vi "Get SLSC Module By Slot.vi"(8 "error in (no error)":errorcluster, 10 "Slot":u32=1, 11 "SLSC Chassis":u64) -> (0 "error out":errorcluster, 2 "SLSC Module":u64, 3 "SLSC Chassis out":u64)   [LabVIEW 2020, in "VeriStand SLSC Scripting.lvlib"]
uses:
  VeriStand SLSC Scripting.lvlib
  NationalInstruments.VeriStand.SystemDefinitionAPI
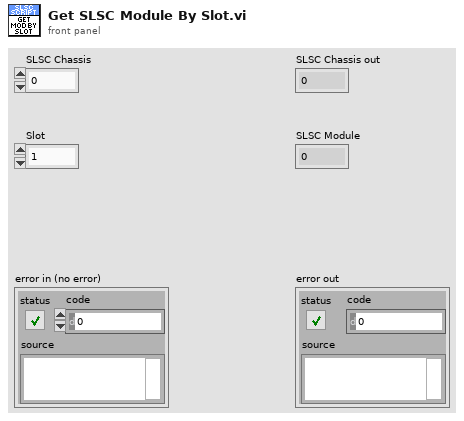
[diagram p1: front panel]
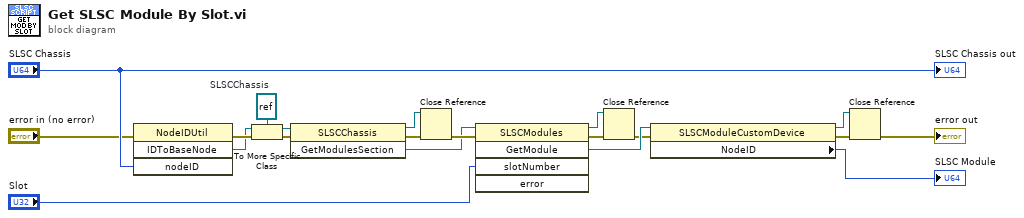
[diagram p0: block diagram]
diagram:
  w14 = refnum<k24> refnum  # SLSCChassis
  n1 = invoke class="NodeIDUtil" method="IDToBaseNode"(error in="error in (no error)", "nodeID"="SLSC Chassis") -> (error out=w11:errorcluster, "IDToBaseNode"=w10:refnum<k24>)  [unwired: 2 in, 2 out]
  n2 = To More Specific Class(target class=w14, reference=w10, error in=w11) -> (specific class reference=w12:refnum<k24>, error out=w13:errorcluster)
  n3 = invoke class="SLSCChassis" method="GetModulesSection"(reference=w12, error in=w13) -> (reference out=w7:refnum<k24>, error out=w9:errorcluster, "GetModulesSection"=w6:refnum<k24>)  [unwired: 1 in]
  n4 = Close Reference(reference=w7, error in (no error)=w9) -> (error out=w18:errorcluster)
  n5 = invoke class="SLSCModules" method="GetModule"(reference=w6, error in=w18, "slotNumber"="Slot") -> (reference out=w1:refnum<k24>, error out=w8:errorcluster, "GetModule"=w4:refnum<k24>)  [unwired: 2 in, 2 out]
  n6 = Close Reference(reference=w1, error in (no error)=w8) -> (error out=w2:errorcluster)
  n7 = property class="SLSCModuleCustomDevice"(reference=w4, error in=w2) -> (reference out=w3:refnum<k24>, error out=w17:errorcluster, "NodeID"=→"SLSC Module":u64)
  n8 = Close Reference(reference=w3, error in (no error)=w17) -> (error out=→"error out":errorcluster)
  "SLSC Chassis out" <- "SLSC Chassis"
